vi "YKMW100 DOE Dishwasher Channel Settings.vi"(8 "Channel_Enum":T1=1 items=["Thermocouple_6", "Water Temperature", "Spare 1", "Water_Pressure", "Unit Weight", "Thermocouple 1", "Thermocouple 2", "Thermocouple 3", "Thermocouple 4", "Thermocouple 5", "Drain Event", "Pump Event", "Water Valve Event", "Heater Event", "Motor Event", "Turbidity Sensor", "Spare 2", "Spare 3", "Spare 4", "Spare 5"]) -> (0 "Channel String":string)   [LabVIEW 2019]
uses:
  Type Definitions/YKMW100 DISH Channel Settings.ctl
panel:
  out "32bit integer":i32
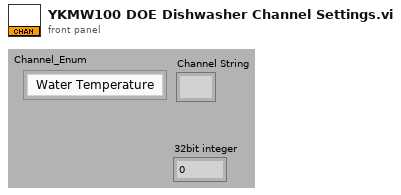
[diagram p1: front panel]
types:
  T1 = typedef "YKMW100 DISH Channel Settings.ctl" = u32
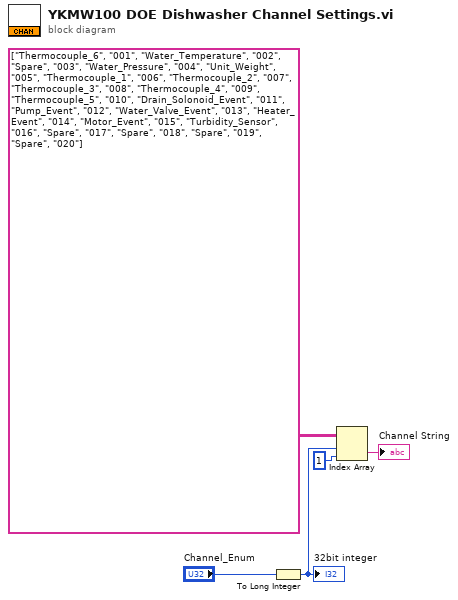
[diagram p0: block diagram]
diagram:
  n1 = To Long Integer(number="Channel_Enum") -> (32bit integer=w3:i32)
  "32bit integer" <- w3
  n2 = Index Array(array=string[][] [["Thermocouple_6", "001"], ["Water_Temperature", "002"], ["Spare", "003"], ["Water_Pressure", "004"], ["Unit_Weight", "005"], ["Thermocouple_1", "006"], ["Thermocouple_2", "007"], ["Thermocouple_3", "008"], ["Thermocouple_4", "009"], ["Thermocouple_5", "010"], ["Drain_Solonoid_Event", "011"], ["Pump_Event", "012"], ["Water_Valve_Event", "013"], ["Heater_Event", "014"], ["Motor_Event", "015"], ["Turbidity_Sensor", "016"], ["Spare", "017"], ["Spare", "018"], ["Spare", "019"], ["Spare", "020"]] ("Sorted 2D Array"), index (row)=w3, index (col)=1 ("disabled index (col)")) -> (element=→"Channel String":string)
